vi "Read Generated Files.vi"(8 "error in (no error)":errorcluster, 11 "Task Outputs in":refnum<class "Task Outputs.lvclass">) -> (0 "error out":errorcluster, 2 "Generated Files":path[](array[path]), 3 "Task Outputs out":refnum<class "Task Outputs.lvclass">)   [LabVIEW 2017, in "Message Interface.lvlib" / "Task Outputs.lvclass"]
uses:
  Task Outputs.lvclass
  Task Outputs.lvclass/Task Outputs.ctl
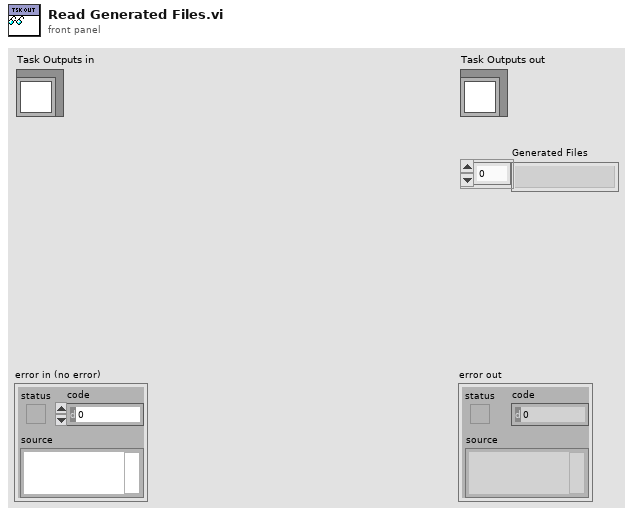
[diagram p1: front panel]
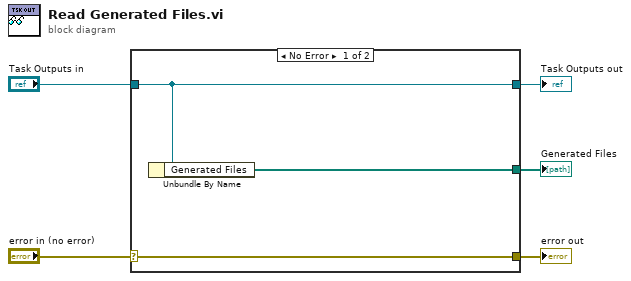
[diagram p0: block diagram]
diagram:
  n1 = case shown="No Error" "error in (no error)" {
    selector: "error in (no error)" -> [w8 w9]
    tunnel: [w8 w9] -> w4
    tunnel: [w7 w10] -> w2
    tunnel: "Task Outputs in" -> [w7 w10]
    tunnel: [w6 _] -> w1
    frame No Error {
      n2 = Unbundle By Name(w7) -> ("Generated Files"=w6:path[])
    }
    frame Error {
    }
  }
  "error out" <- w4
  "Task Outputs out" <- w2
  "Generated Files" <- w1
